vi "StopContinuous.vi"(8 "error in (no error)":errorcluster, 11 "config":T1) -> (0 "error out":errorcluster, 3 "config out":T1)   [LabVIEW 2017, in "EmsaAcquisition.lvlib"]
uses:
  <vilib>/addons/InsightCM/Devices/Shared/Emsa/EmsaAcquisition/EmsaAcquisition.lvlib
  <vilib>/addons/InsightCM/Devices/Shared/Emsa/EmsaAcquisition/controls/config.ctl
  <vilib>/addons/InsightCM/Devices/Shared/Emsa/Emsa9770API/9770 API.lvclass
  <vilib>/addons/InsightCM/Devices/Shared/Emsa/EmsaAcquisition/controls/group.ctl
  <vilib>/addons/InsightCM/Devices/Shared/Emsa/EmsaAcquisition/controls/acqConfig.ctl
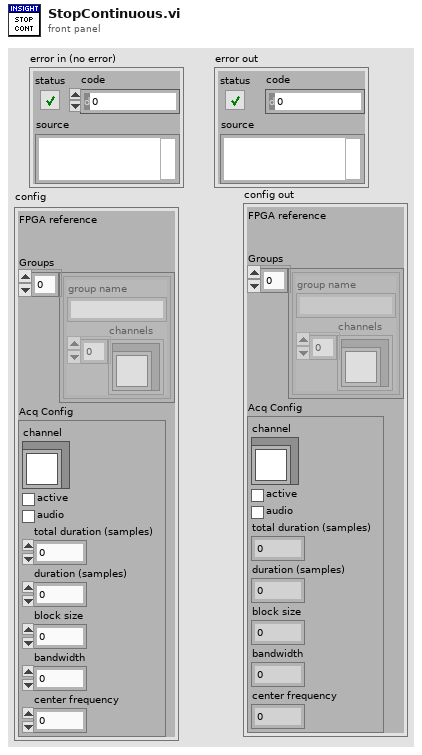
[diagram p1: front panel]
types:
  T1 = typedef "EmsaAcquisition.lvlib/config.ctl" = cluster{"FPGA reference":refnum<k20>, "Groups":T2[], "Acq Config":T3}
  T2 = typedef "EmsaAcquisition.lvlib/group.ctl" = cluster{"group name":string, "channels":refnum<class "9770 API.lvclass">[]}
  T3 = typedef "EmsaAcquisition.lvlib/acqConfig.ctl" = cluster{"channel":refnum<class "9770 API.lvclass">, "active":bool, "audio":bool, "total duration (samples)":i32, "duration (samples)":i32, "block size":i32, "bandwidth":dbl, "center frequency":dbl}
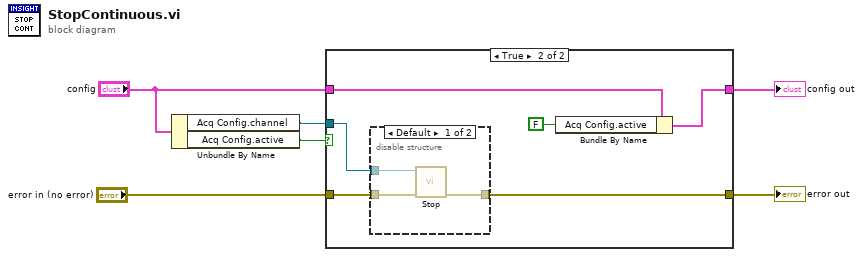
[diagram p0: block diagram]
diagram:
  n1 = Unbundle By Name("config") -> ("Acq Config.channel"=w3:refnum<class "9770 API.lvclass">, "Acq Config.active"=w6:bool)
  n2 = case shown="True" w6 {
    tunnel: w3 -> [_ w14]
    tunnel: "error in (no error)" -> [w8 w13]
    tunnel: [w8 w12] -> w5
    tunnel: "config" -> [w7 w11]
    tunnel: [w7 w9] -> w1
    frame False {
    }
    frame True {
      n3 = disable-structure shown="Default" {
        disable-tunnel: w14 -> [w17 _]
        disable-tunnel: w13 -> [w16 w18]
        disable-tunnel: [w15 w18] -> w12
        frame condition #0 {
          n4 = call-dynamic "Stop.vi"("error in (no error)"=w16, "RIO_API in"=w17) -> ("error out"=w15:errorcluster)  [unwired: 8 in, 1 out]
        }
        frame condition #1 (active) {
        }
      }
      n5 = Bundle By Name(cluster=w11, "Acq Config.active"=FALSE ("active")) -> (w9:T1)
    }
  }
  "error out" <- w5
  "config out" <- w1
